vi "复制vi.vi"() -> ()   [LabVIEW 2014]
panel:
  in  "数值":i32=7
  in  "路径":path=path "C:/Users/chen/Desktop/onedrive/3-Evehicle/activity/module1Activity.vi"
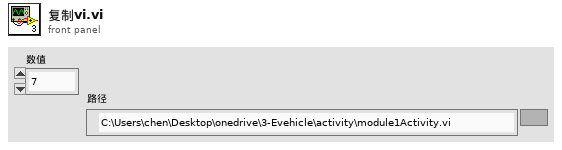
[diagram p1: front panel]
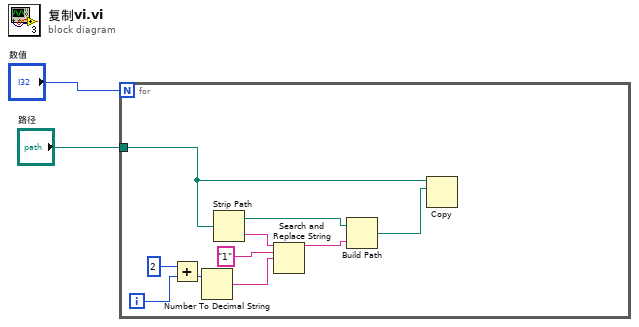
[diagram p0: block diagram]
diagram:
  n1 = for {
    N: "数值" -> [_]
    tunnel: "路径" -> [w12]
    i -> [w9]
    n2 = Add(x=2, y=w9) -> (x+y=w4:i32)
    n3 = Number To Decimal String(number=w4) -> (decimal integer string=w8:string)  [unwired: 1 in]
    n4 = Strip Path(path=w12) -> (stripped path=w7:path, name=w11:string)
    n5 = Search and Replace String(input string=w11, search string="1" ("搜索字符串"), replace string=w8) -> (result string=w6:string)  [unwired: 5 in, 3 out]
    n6 = Build Path(base path=w7, name or relative path=w6) -> (appended path=w5:path)
    n7 = Copy(10:w5, 11:w12) -> ()  [unwired: 3 in, 3 out]
  }
